vi "LB_ItemIndex_Tests.vi"(11 "error in":errorcluster) -> (15 "error out":errorcluster)   [LabVIEW 2016, in "DronaTest.lvlib"]
uses:
  DronaTest.lvlib
  APIs/Stimulus/ControlValue/SetValueAuto.vi
  APIs/Stimulus/ControlValue/Controls/Listbox/SetValueByItemIndex.vi
  APIs/Assert/AssertControlValue/Equal.vi
  <vilib>/addons/_JKI Toolkits/Caraya/classes/Assert/Assert Error.vi
  <vilib>/addons/_JKI Toolkits/Caraya/classes/Test/Test.lvclass
  Drona.lvlib
  <vilib>/SLL Toolkit/SLL Debug/SLL Debug.lvlib
  APIs/Stimulus/ControlValue/Controls/Listbox/StimulusListbox.lvlib
  APIs/Assert/AssertControlValue/AssertControlValue.lvlib
  APIs/Stimulus/ControlValue/ControlValue.lvlib
  <vilib>/addons/_JKI Toolkits/Caraya/classes/Assert/Assert.lvclass
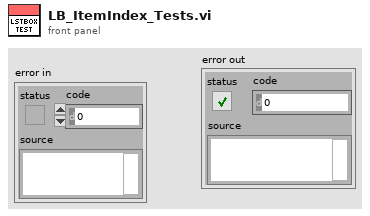
[diagram p1: front panel]
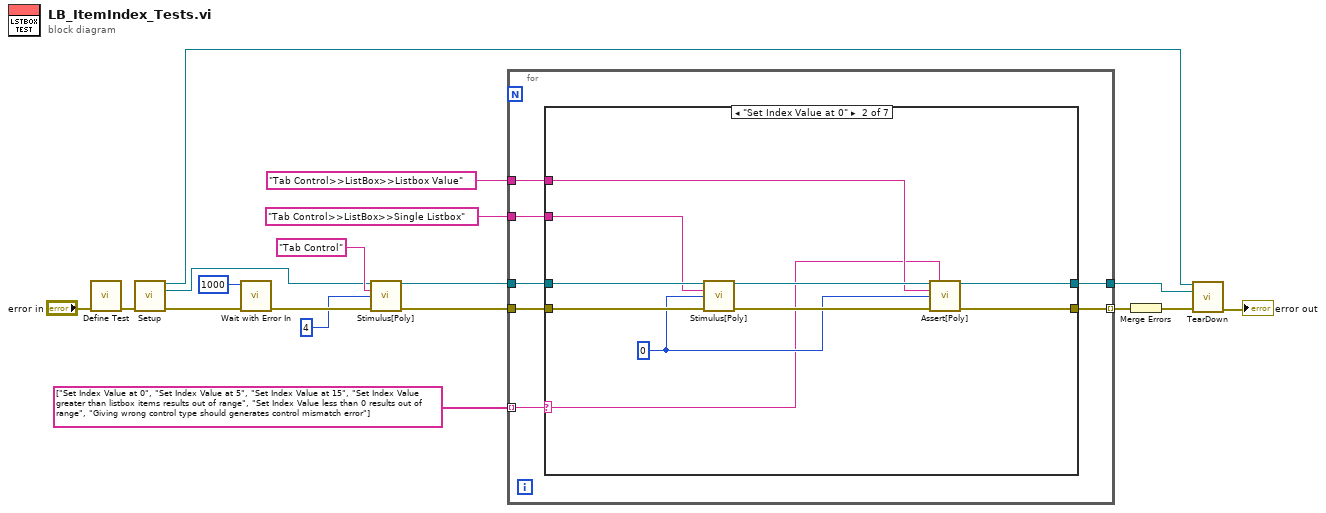
[diagram p0: block diagram]
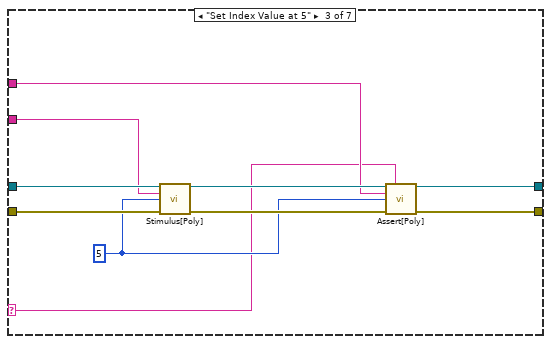
[diagram p3: hidden frame]
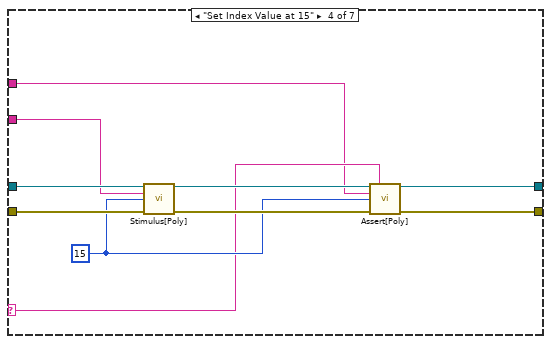
[diagram p4: hidden frame]
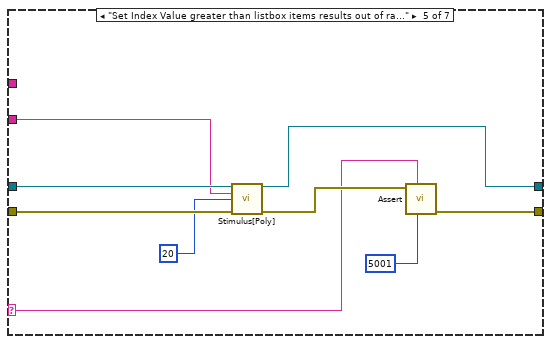
[diagram p5: hidden frame]
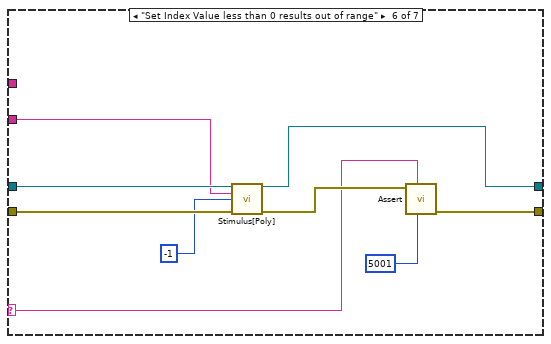
[diagram p6: hidden frame]
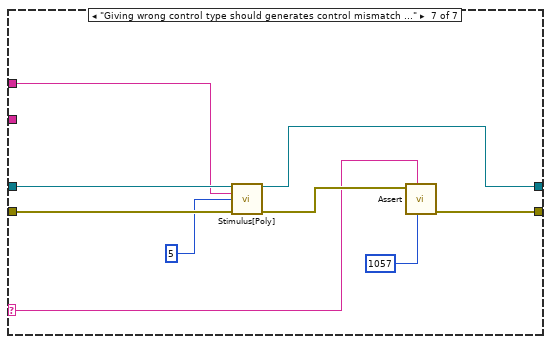
[diagram p7: hidden frame]
diagram:
  n1 = call <vilib>:"Define Test.vi"("error in (no error)"="error in") -> ("error out"=w7:errorcluster)  [unwired: 9 in, 1 out]
  n2 = call "Setup.vi"("error in (no error)"=w7) -> ("Application Ref"=w3:refnum<vi>, "VI out"=w5:refnum<vi>, "error out"=w6:errorcluster)  [unwired: 12 in]
  n3 = call <vilib>:"Wait with Error In.vi"("error in (no error)"=w6, "milliseconds to wait"=u32 1000) -> ("error out"=w16:errorcluster)  [unwired: 9 in]
  n4 = call-poly "Stimulus[Poly].vi"("VI Reference In"=w5, "Control Path"="Tab Control", "Value (Signaling)"=4, "error in"=w16) -> ("VI Reference Out"=w12:refnum<vi>, "error out"=w15:errorcluster)  [unwired: 10 in]
  n5 = for {
    tunnel: w12 -> [w24]
    tunnel: "Tab Control>>ListBox>>Single Listbox" ("Control Path") -> [w23]
    tunnel: "Tab Control>>ListBox>>Listbox Value" ("Control Path") -> [w22]
    tunnel: string[] ["Set Index Value at 0", "Set Index Value at 5", "Set Index Value at 15", "Set Index Value greater than listbox items results out of range", "Set Index Value less than 0 results out of range", "Giving wrong control type should generates control mismatch error"] -> [w20] mode=indexing
    tunnel: [w19] -> w2
    tunnel: w15 -> [w25]
    tunnel: [w21] -> w8 mode=indexing
    n6 = case shown="\"Set Index Value at 0\"" w20 {
      selector: w20 -> [_ w28 w38 w50 w60 w69 w79]
      tunnel: w25 -> [w27 w37 w47 w57 w66 w75 w84]
      tunnel: w24 -> [w26 w36 w46 w56 w65 w74 w83]
      tunnel: w23 -> [_ w32 w42 w48 w63 w72 _]
      tunnel: w22 -> [_ w31 w41 w49 _ _ w76]
      tunnel: [w27 w30 w40 w52 w61 w70 w80] -> w21
      tunnel: [w26 w29 w39 w51 w58 w67 w77] -> w19
      frame Default {
      }
      frame "Set Index Value at 0" {
        w33 = 0 ("Item Index")
        n7 = call-poly "Stimulus[Poly].vi"("VI Reference In"=w36, "Control Path"=w32, "Item Index"=w33, "Error In"=w37) -> ("VI Reference Out"=w34:refnum<vi>, "Error Out"=w35:errorcluster)  [unwired: 10 in]
        n8 = call-poly "Assert[Poly].vi"("VI Reference In"=w34, "Test Label"=w28, "Control Path"=w31, "Control Value"=w33, "Error In"=w35) -> ("VI Reference Out"=w29:refnum<vi>, "Error Out"=w30:errorcluster)  [unwired: 8 in, 1 out]
      }
      frame "Set Index Value at 5" {
        w43 = 5 ("Item Index")
        n9 = call-poly "Stimulus[Poly].vi"("VI Reference In"=w46, "Control Path"=w42, "Item Index"=w43, "Error In"=w47) -> ("VI Reference Out"=w44:refnum<vi>, "Error Out"=w45:errorcluster)  [unwired: 10 in]
        n10 = call-poly "Assert[Poly].vi"("VI Reference In"=w44, "Test Label"=w38, "Control Path"=w41, "Control Value"=w43, "Error In"=w45) -> ("VI Reference Out"=w39:refnum<vi>, "Error Out"=w40:errorcluster)  [unwired: 8 in, 1 out]
      }
      frame "Set Index Value at 15" {
        w53 = 15 ("Item Index")
        n11 = call-poly "Stimulus[Poly].vi"("VI Reference In"=w56, "Control Path"=w48, "Item Index"=w53, "Error In"=w57) -> ("VI Reference Out"=w54:refnum<vi>, "Error Out"=w55:errorcluster)  [unwired: 10 in]
        n12 = call-poly "Assert[Poly].vi"("VI Reference In"=w54, "Test Label"=w50, "Control Path"=w49, "Control Value"=w53, "Error In"=w55) -> ("VI Reference Out"=w51:refnum<vi>, "Error Out"=w52:errorcluster)  [unwired: 8 in, 1 out]
      }
      frame "Set Index Value greater than listbox items results out of range" {
        n13 = call-poly "Stimulus[Poly].vi"("VI Reference In"=w65, "Control Path"=w63, "Item Index"=20, "Error In"=w66) -> ("VI Reference Out"=w58:refnum<vi>, "Error Out"=w62:errorcluster)  [unwired: 10 in]
        n14 = call-poly <vilib>:"Assert.vi"("error code (1)"=5001, "Label"=w60, "Error?"=w62) -> ("error out"=w61:errorcluster)  [unwired: 7 in, 1 out]
      }
      frame "Set Index Value less than 0 results out of range" {
        n15 = call-poly "Stimulus[Poly].vi"("VI Reference In"=w74, "Control Path"=w72, "Item Index"=-1, "Error In"=w75) -> ("VI Reference Out"=w67:refnum<vi>, "Error Out"=w71:errorcluster)  [unwired: 10 in]
        n16 = call-poly <vilib>:"Assert.vi"("error code (1)"=5001, "Label"=w69, "Error?"=w71) -> ("error out"=w70:errorcluster)  [unwired: 7 in, 1 out]
      }
      frame "Giving wrong control type should generates control mismatch error" {
        n17 = call-poly "Stimulus[Poly].vi"("VI Reference In"=w83, "Control Path"=w76, "Item Index"=5, "Error In"=w84) -> ("VI Reference Out"=w77:refnum<vi>, "Error Out"=w81:errorcluster)  [unwired: 10 in]
        n18 = call-poly <vilib>:"Assert.vi"("error code (1)"=1057, "Label"=w79, "Error?"=w81) -> ("error out"=w80:errorcluster)  [unwired: 7 in, 1 out]
      }
    }
  }
  n19 = Merge Errors(w8) -> (w4:errorcluster)
  n20 = call "TearDown.vi"("Application Ref"=w3, "VI in"=w2, "error in (no error)"=w4) -> ("error out"=→"error out":errorcluster)  [unwired: 12 in]
